vi "Symphony Acquire Image.vi"(5 "Noise Mode":T1=enum."One For All Acq", 6 "AcqBusy":refnum<vi>, 7 "ImageMode":bool, 8 "error in":errorcluster caption="entrée d'erreur (pas d'erreur)", 9 "Accumulations":u16=1 min=1 step=1, 10 "ShutterEnable":bool, 11 "JYCCDLib.IJYCCDReqd":refnum<k7>) -> (0 "error out":errorcluster, 1 "Acq Time(ms)":u32, 2 "AcquisitionBusy":bool, 3 "Datas":i32[][][](array[numeric]))   [LabVIEW 2019]
uses:
  NoiseCorr.ctl
  Symphony Acq Image States.ctl
  <vilib>/Utility/error.llb/DialogType.ctl
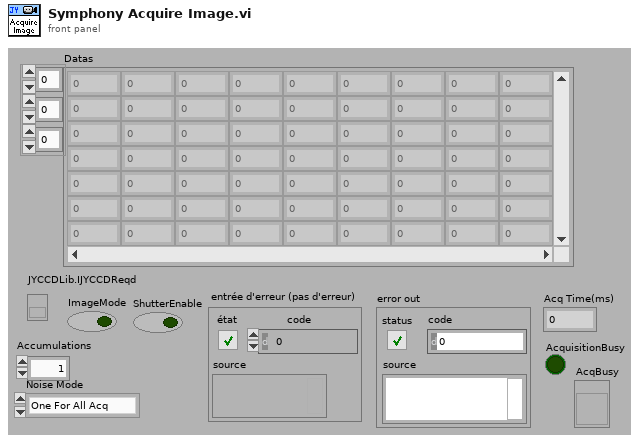
[diagram p1: front panel]
types:
  T1 = typedef "NoiseCorr.ctl" = enum16{"Off", "One For All Acq", "One For Every Acq"}
  T2 = typedef "Symphony Acq Image States.ctl" = enum16{"Start Acq", "Acq Busy", "ReqData", "GetDataObj", "AcqDone", "Error"}
  T3 = typedef "DialogType.ctl" = u16
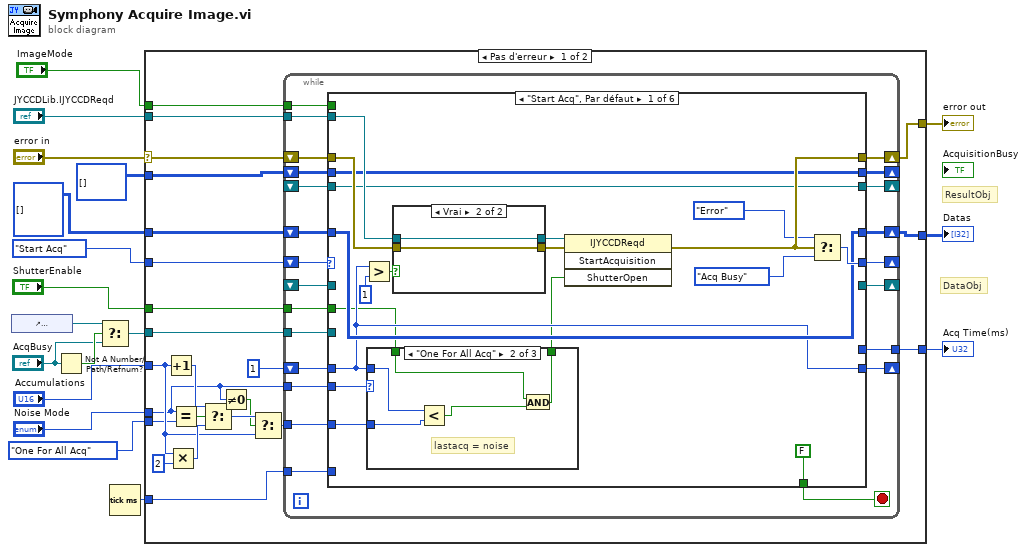
[diagram p0: block diagram]
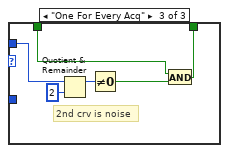
[diagram p3: hidden frame]
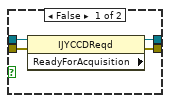
[diagram p4: hidden frame]
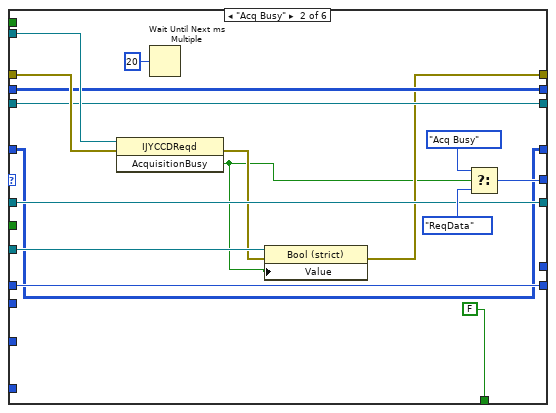
[diagram p5: hidden frame]
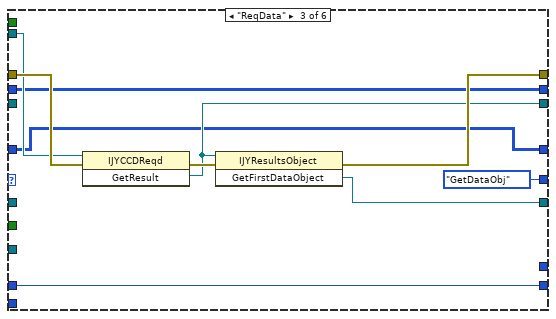
[diagram p6: hidden frame]
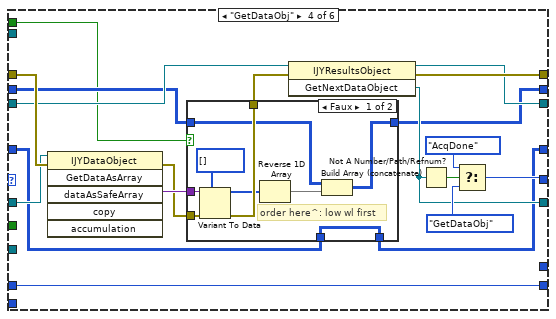
[diagram p7: hidden frame]
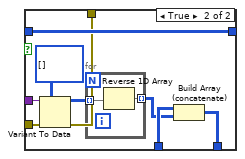
[diagram p8: hidden frame]
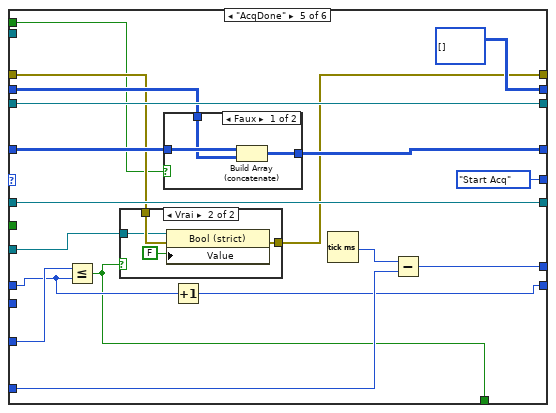
[diagram p9: hidden frame]
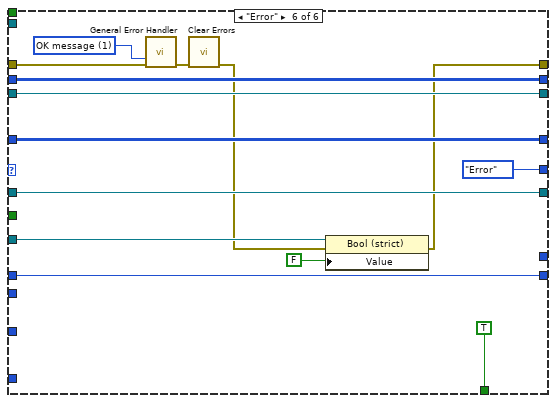
[diagram p12: hidden frame]
diagram:
  # "DataObj"
  # "ResultObj"
  n1 = control-ref of="AcquisitionBusy"() -> (w6:refnum<vi>)
  n2 = Not A Number/Path/Refnum?(number/path/refnum="AcqBusy") -> (NaN/Path/Refnum?=w7:bool)
  n3 = Select(t=w6, s=w7, f="AcqBusy") -> (s? t:f=w4:refnum<vi>)
  n4 = Tick Count (ms)() -> (millisecond timer value=w16:u32)
  n5 = case shown="Pas d'erreur" "error in" {
    selector: "error in" -> [w40 w208]
    tunnel: "JYCCDLib.IJYCCDReqd" -> [w41 _]
    tunnel: [w35 _] -> w18
    tunnel: w16 -> [w39 _]
    tunnel: Symphony_Acq_Image_States."Start Acq" -> [w38 _]
    tunnel: "ShutterEnable" -> [w37 _]
    tunnel: i32[][][] [] ("type") -> [w36 _]
    tunnel: [w34 _] -> w12
    tunnel: "Accumulations" -> [w24 _]
    tunnel: [w33 w208] -> w10
    tunnel: i32[][] [] ("type") -> [w32 _]
    tunnel: w4 -> [w31 _]
    tunnel: "ImageMode" -> [w30 _]
    tunnel: "Noise Mode" -> [w20 _]
    tunnel: NoiseCorr."One For All Acq" ("Noise Mode") -> [w21 _]
    frame No Error {
      n6 = Increment(x=w24) -> (x+1=w26:u16)
      n7 = Multiply(x=w24, y=u16 2) -> (x*y=w27:u16)
      n8 = Equal?(x=w20, y=w21) -> (x = y?=w22:bool)
      n9 = Select(t=w26, s=w22, f=w27) -> (s? t:f=w25:u16)
      n10 = Not Equal To 0?(x=w20) -> (x != 0?=w19:bool)
      n11 = Select(t=w25, s=w19, f=w24) -> (s? t:f=w23:u16)
      n12 = while {
        tunnel: w41 -> [w61]
        tunnel: w39 -> [w63]
        shift-right: [w57] -> _
        shift-left: w38 -> [w62]
        shift-right: [w59] -> w33
        shift-left: w40 -> [w60]
        tunnel: w37 -> [w58]
        shift-right: [w56] -> _
        shift-left: _ -> [w52]
        shift-right: [w55] -> _
        shift-left: _ -> [w54]
        shift-right: [w64] -> w35
        shift-left: w36 -> [w53]
        tunnel: [w50] -> w34
        tunnel: w23 -> [w49]
        shift-right: [w47] -> _
        shift-left: u16 1 ("Accumulations:") -> [w48]
        shift-right: [w45] -> _
        shift-left: w32 -> [w46]
        tunnel: w31 -> [w44]
        tunnel: w30 -> [w43]
        tunnel: w20 -> [w42]
        stop <- w51 stop-if-true
        n13 = case shown="\"Start Acq\", Par défaut" w62 {
          tunnel: [w70 w102 w118 w128 w174 w206] -> w64
          tunnel: w63 -> [_ _ _ _ w183 _]
          tunnel: w61 -> [w81 w117 w125 _ _ _]
          tunnel: w60 -> [w80 w116 w127 w146 w170 w203]
          tunnel: [w79 w104 w124 w143 w169 w195] -> w59
          tunnel: w58 -> [w67 _ _ _ _ _]
          tunnel: [w76 w114 Symphony_Acq_Image_States."GetDataObj" w139 Symphony_Acq_Image_States."Start Acq" Symphony_Acq_Image_States."Error"] -> w57
          tunnel: [w72 w109 w123 w137 w177 w205] -> w56
          tunnel: [_ w108 w122 w136 w176 w204] -> w55
          tunnel: w54 -> [_ w108 _ w145 w176 w204]
          tunnel: w53 -> [w70 w102 w118 w129 w173 w206]
          tunnel: w52 -> [w72 w109 _ w144 w177 w205]
          tunnel: [FALSE FALSE _ _ w171 TRUE] -> w51
          tunnel: [_ _ _ _ w182 _] -> w50
          tunnel: w49 -> [w69 _ _ _ w180 _]
          tunnel: w48 -> [w68 w110 w120 w138 w179 w199]
          tunnel: [w68 w110 w120 w138 w178 w199] -> w47
          tunnel: w46 -> [w71 w107 w119 w134 w172 w198]
          tunnel: [w71 w107 w119 w135 i32[][] [] w198] -> w45
          tunnel: w44 -> [_ w106 _ _ w168 w197]
          tunnel: w43 -> [_ _ _ w130 w167 _]
          tunnel: w42 -> [w65 _ _ _ _ _]
          frame "Start Acq", Default {
            n14 = Greater?(x=w68, y=u16 1) -> (0:w74:bool)
            n15 = case shown="\"One For All Acq\"" w65 {
              tunnel: w69 -> [_ w89 _]
              tunnel: w68 -> [_ w88 w95]
              tunnel: w67 -> [w84 w85 w92]
              tunnel: [w84 w87 w94] -> w66
              frame "Off", Default {
              }
              frame "One For All Acq" {
                # "lastacq = noise"
                n16 = Less?(x=w88, y=w89) -> (x < y?=w86:bool)
                n17 = And(x=w85, y=w86) -> (x .and. y?=w87:bool)
              }
              frame "One For Every Acq" {
                # "2nd crv is noise"
                n18 = Quotient & Remainder(x=w95, y=u16 2) -> (x-y*floor(x/y)=w90:u16)  [unwired: 1 out]
                n19 = Not Equal To 0?(x=w90) -> (x != 0?=w93:bool)
                n20 = And(x=w92, y=w93) -> (x .and. y?=w94:bool)
              }
            }
            n21 = case shown="Vrai" w74 {
              tunnel: [w99 w101] -> w83
              tunnel: [w98 w100] -> w82
              tunnel: w81 -> [w97 w101]
              tunnel: w80 -> [w96 w100]
              frame False {
                n22 = property class="IJYCCDReqd" props=["ReadyForAcquisition"](reference=w97, error in=w96) -> (reference out=w99:refnum<k7>, error out=w98:errorcluster)  [unwired: 1 out]
              }
              frame True {
              }
            }
            n23 = invoke class="IJYCCDReqd" method="StartAcquisition"(reference=w83, error in=w82, "ShutterOpen"=w66) -> (error out=w79:errorcluster)  [unwired: 1 in, 3 out]
            n24 = Select(t=Symphony_Acq_Image_States."Error", s=w79, f=Symphony_Acq_Image_States."Acq Busy") -> (s? t:f=w76:T2)
          }
          frame "Acq Busy" {
            n25 = invoke class="IJYCCDReqd" method="AcquisitionBusy"(reference=w117, error in=w116) -> (error out=w105:errorcluster, "AcquisitionBusy"=w103:bool)  [unwired: 1 in, 1 out]
            n26 = Wait Until Next ms Multiple(millisecond multiple=u32 20 ("n millisecondes")) -> ()  [unwired: 1 out]
            n27 = property class="Bool (strict)"(reference=w106, error in=w105, "Value"=w103) -> (error out=w104:errorcluster)  [unwired: 1 out]
            n28 = Select(t=Symphony_Acq_Image_States."Acq Busy", s=w103, f=Symphony_Acq_Image_States."ReqData") -> (s? t:f=w114:T2)
          }
          frame "ReqData" {
            n29 = invoke class="IJYCCDReqd" method="GetResult"(reference=w125, error in=w127) -> (error out=w126:errorcluster, "GetResult"=w123:refnum<k7>)  [unwired: 1 in, 1 out]
            n30 = invoke class="IJYResultsObject" method="GetFirstDataObject"(reference=w123, error in=w126) -> (error out=w124:errorcluster, "GetFirstDataObject"=w122:refnum<k7>)  [unwired: 1 in, 1 out]
          }
          frame "GetDataObj" {
            n31 = invoke class="IJYDataObject" method="GetDataAsArray"(reference=w145, error in=w146) -> (error out=w132:errorcluster, "dataAsSafeArray"=w133:variant)  [unwired: 4 in, 4 out]
            n32 = case shown="Faux" w130 {
              tunnel: w134 -> [w150 w164]
              tunnel: [w155 w164] -> w135
              tunnel: w133 -> [w153 w163]
              tunnel: w132 -> [w152 w162]
              tunnel: [w151 w160] -> w131
              tunnel: w129 -> [w148 w159]
              tunnel: [w148 w158] -> w128
              frame False {
                # "order here^: low wl first"
                n33 = Variant To Data(error in=w152, type=i32[] [], Variant=w153) -> (data=w149:i32[], error out=w151:errorcluster)
                n34 = Reverse 1D Array(array=w149) -> (reversed array=w147:i32[])
                n35 = Build Array (concatenate)(w150, w147) -> (w155:i32[][])
              }
              frame True {
                n36 = Variant To Data(error in=w162, type=i32[][] [], Variant=w163) -> (data=w157:i32[][], error out=w160:errorcluster)
                n37 = for {
                  tunnel: w157 -> [w166] mode=indexing
                  tunnel: [w165] -> w156 mode=indexing
                  n38 = Reverse 1D Array(array=w166) -> (reversed array=w165:i32[])
                }
                n39 = Build Array (concatenate)(w159, w156) -> (w158:i32[][][])
              }
            }
            n40 = invoke class="IJYResultsObject" method="GetNextDataObject"(reference=w144, error in=w131) -> (reference out=w137:refnum<k7>, error out=w143:errorcluster, "GetNextDataObject"=w136:refnum<k7>)  [unwired: 1 in]
            n41 = Not A Number/Path/Refnum?(number/path/refnum=w136) -> (NaN/Path/Refnum?=w142:bool)
            n42 = Select(t=Symphony_Acq_Image_States."AcqDone", s=w142, f=Symphony_Acq_Image_States."GetDataObj") -> (s? t:f=w139:T2)
          }
          frame "AcqDone" {
            n43 = Less Or Equal?(x=w180, y=w179) -> (x <= y?=w171:bool)
            n44 = case shown="Vrai" w171 {
              tunnel: w170 -> [w189 w193]
              tunnel: [w189 w192] -> w169
              tunnel: w168 -> [_ w191]
              frame False {
              }
              frame True {
                n45 = property class="Bool (strict)"(reference=w191, error in=w193, "Value"=FALSE) -> (error out=w192:errorcluster)  [unwired: 1 out]
              }
            }
            n46 = case shown="Faux" w167 {
              tunnel: [w187 w188] -> w174
              tunnel: w173 -> [w186 w188]
              tunnel: w172 -> [w185 _]
              frame False {
                n47 = Build Array (concatenate)(w186, w185) -> (w187:i32[][][])
              }
              frame True {
              }
            }
            n48 = Increment(x=w179) -> (x+1=w178:u16)
            n49 = Tick Count (ms)() -> (millisecond timer value=w184:u32)
            n50 = Subtract(x=w184, y=w183) -> (x-y=w182:u32)
          }
          frame "Error" {
            w201 = T3 1 items=["no dialog", "OK message", "continue or stop message", "OK message + warnings", "continue/stop + warnings"] ("type of dialog (OK msg:1)")
            n51 = call <vilib>:"General Error Handler.vi"("type of dialog (OK msg:1)"=w201, "error in (no error)"=w203) -> ("error out"=w202:errorcluster)  [unwired: 9 in, 4 out]
            n52 = call <vilib>:"Clear Errors.vi"("error in (no error)"=w202) -> ("error out"=w196:errorcluster)  [unwired: 5 in, 1 out]
            n53 = property class="Bool (strict)"(reference=w197, error in=w196, "Value"=FALSE) -> (error out=w195:errorcluster)  [unwired: 1 out]
          }
        }
      }
    }
    frame Error {
    }
  }
  "Datas" <- w18
  "Acq Time(ms)" <- w12
  "error out" <- w10
